vi "Actor Core.vi"(8 "error in":errorcluster, 11 "Data Logger in":refnum<class "Data Logger.lvclass">) -> (0 "error out":errorcluster, 3 "Actor out":refnum<class "Actor.lvclass">)   [LabVIEW 2017, in "Data Logger.lvlib" / "Data Logger.lvclass"]
doc: "(<B>Filename</B>: Actor Framework.lvlib:Actor.lvclass:Actor Core.vi)\n\nReceives messages to the actor, reacts to them, and initiates any error handling that may shut the actor down.\n\nDescendant classes may override this VI to append parallel tasks for the actor to complete while it handles messages. Overrides use the Call Parent Method node."
uses:
  Data Logger.lvclass
  C:/Program Files (x86)/National Instruments/LabVIEW 2017/vi.lib/ActorFramework/Actor/Actor.lvclass
  <vilib>/ActorFramework/Actor/Actor.lvclass
  <vilib>/ActorFramework/Actor/Actor.lvclass/Actor.ctl
  <vilib>/ActorFramework/Message Enqueuer/Message Enqueuer.lvclass/Message Enqueuer.ctl
  Data Logger Messages/initialize Msg/initialize Msg.lvclass/initialize Msg.ctl
  <vilib>/ActorFramework/Message Enqueuer/Init from Existing Queue.vi
  <vilib>/ActorFramework/Message Enqueuer/Enqueue.vi
  Data Logger Messages/initialize Msg/initialize Msg.lvclass
  C:/Program Files (x86)/National Instruments/LabVIEW 2017/vi.lib/ActorFramework/Message/Message.lvclass
  <vilib>/ActorFramework/Message Priority Queue/Priority Enqueue.vi
  <vilib>/ActorFramework/Message Enqueuer/Message Enqueuer.lvclass
panel:
  in  "file path (use dialog)":path
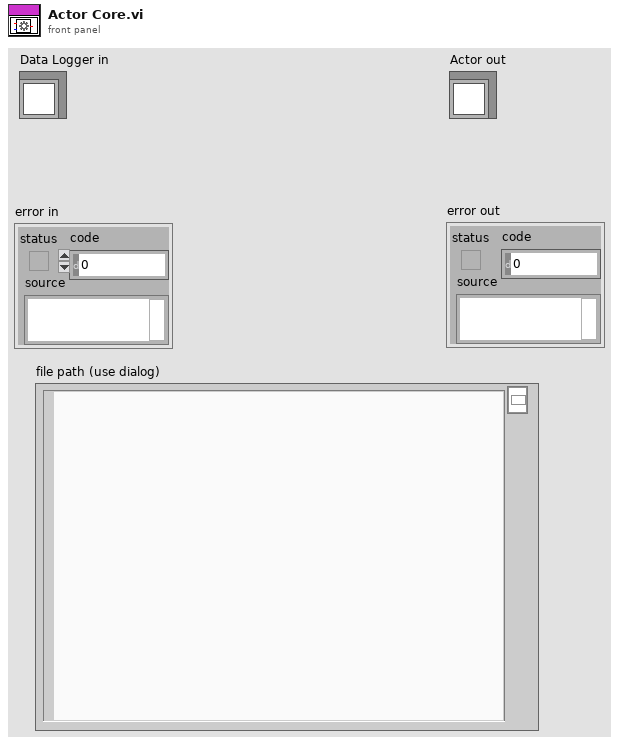
[diagram p1: front panel]
types:
  T1 = enum32{"Invalid", "Standard", "Closed", "Hidden", "Minimized", "Maximized"}
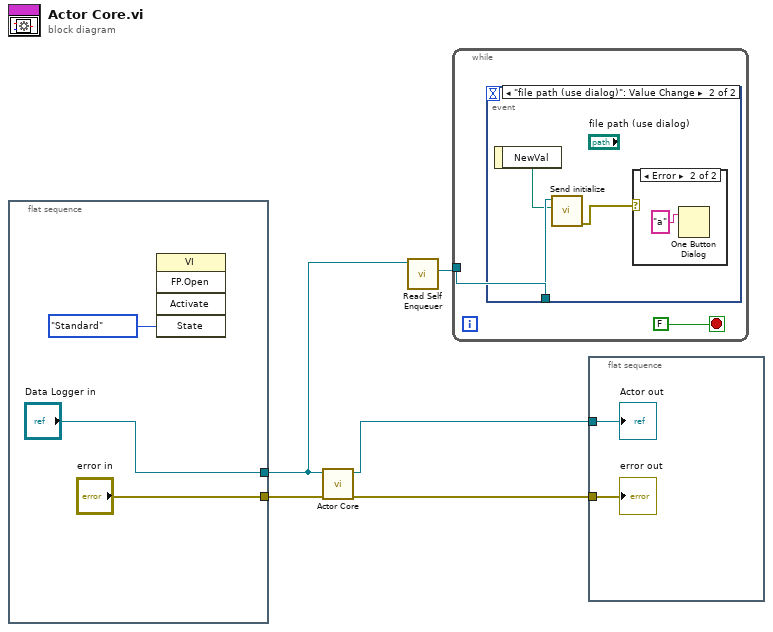
[diagram p0: block diagram]
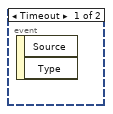
[diagram p2: hidden frame]
diagram:
  n1 = flat-sequence {
    tunnel: ["error in"] -> w3
    tunnel: ["Data Logger in"] -> w2
    frame #0 {
      n2 = invoke class="VI" method="FP.Open"("State"=T1."Standard") -> ()  [unwired: 4 in, 5 out]
    }
  }
  n3 = call-parent "Actor Core.vi"("error in"=w3, "Actor in"=w2) -> ("error out"=w5:errorcluster, "Actor out"=w4:refnum<class "Actor.lvclass">)  [unwired: 8 in]
  n4 = call <vilib>:"Read Self Enqueuer.vi"("Actor"=w2) -> ("Self Enqueuer"=w1:refnum<class "Message Enqueuer.lvclass">)  [unwired: 10 in]
  n5 = while {
    tunnel: w1 -> [w9]
    stop <- FALSE stop-if-true
    n6 = event shown="[1] \"file path (use dialog)\": Value Change" {
      selector: _ -> [_ _]
      dyn-events: _ -> [_ _]
      timeout: _ -> [_ _]
      tunnel: w9 -> [_ w13]
      event Timeout {
        n7 = event-data() -> ()  [unwired: 1 in, 2 out]
      }
      event "file path (use dialog)": Value Change {
        n8 = event-data() -> ("NewVal"=w12:path)  [unwired: 1 in]
        n9 = call "Send initialize.vi"("file path (use dialog)"=w12, "Message Enqueuer"=w13) -> ("error out"=w11:errorcluster)  [unwired: 8 in, 1 out]
        n10 = case shown="Error" w11 {
          frame No Error {
          }
          frame Error {
            n11 = One Button Dialog(message="a") -> ()  [unwired: 1 in, 1 out]
          }
        }
      }
    }
  }
  n12 = flat-sequence {
    tunnel: w5 -> [w16]
    tunnel: w4 -> [w15]
    frame #0 {
      "error out" <- w16
      "Actor out" <- w15
    }
  }
